vi "Read.vi"(6 "Timeout ms (1000)":i32=1000, 8 "Error In":errorcluster, 11 "Receiver Ref.":refnum<class "Receiver.lvclass">) -> (0 "Error Out":errorcluster, 1 "Received?":bool, 2 "Value":variant, 3 "Receiver Ref.":refnum<class "Receiver.lvclass">)   [LabVIEW 2020, in "RemoteVariables.lvlib" / "Receiver.lvclass"]
uses:
  Receiver.lvclass
  Receiver.lvclass/Receiver.ctl
  RawData.ctl
  RemoteVariables.lvlib
  UDP/UDP.lvclass
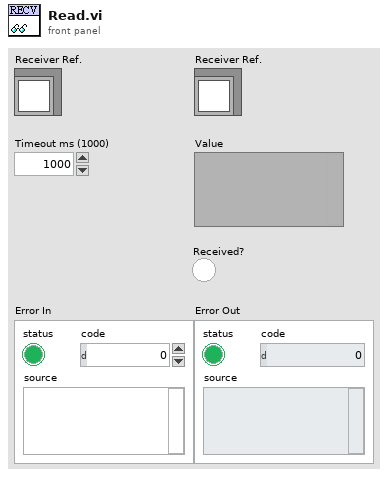
[diagram p1: front panel]
types:
  T1 = typedef "RemoteVariables.lvlib/RawData.ctl" = cluster{"Type string":i16[], "Data string":string}
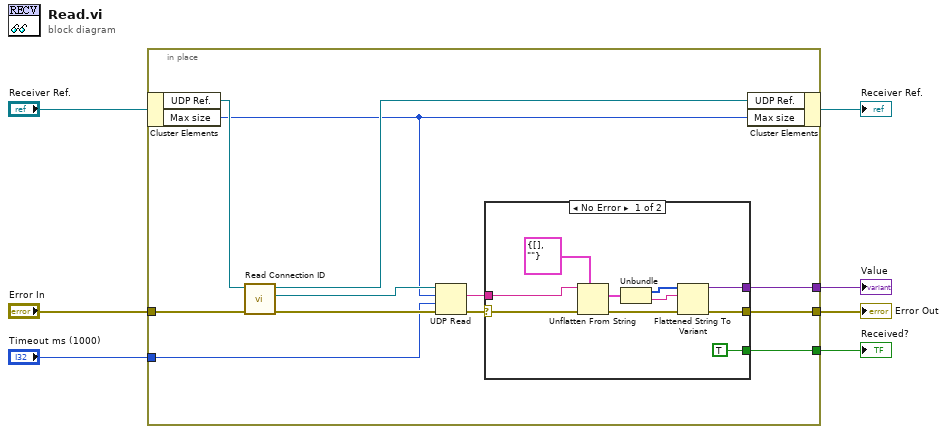
[diagram p0: block diagram]
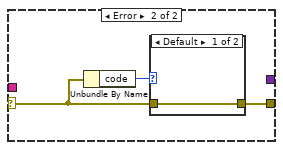
[diagram p2: hidden frame]
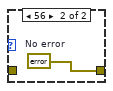
[diagram p3: hidden frame]
diagram:
  n1 = in-place {
    in-place-border: "Timeout ms (1000)" -> [w18]
    in-place-border: [w17] -> w6
    in-place-border: [w16] -> w5
    in-place-border: [w15] -> w4
    in-place-border: "Error In" -> [w12]
    n2 = in-place-cluster #1("Receiver Ref.") -> ("UDP Ref."=w10:refnum<class "UDP.lvclass">, "Max size"=w8:i32)
    n3 = call "Read Connection ID.vi"("error in (no error)"=w12, "UDP in"=w10) -> ("error out"=w19:errorcluster, "UDP Connection ID"=w11:refnum<k16>, "UDP out"=w9:refnum<class "UDP.lvclass">)  [unwired: 7 in]
    n4 = UDP Read(connection ID=w11, max size (548)=w8, timeout ms (25000)=w18, 8:w19) -> (data out=w13:string, error out=w14:errorcluster)  [unwired: 3 out]
    n5 = case shown="No Error" w14 {
      selector: w14 -> [w29 w31]
      tunnel: w13 -> [w28 _]
      tunnel: [w22 w30] -> w17
      tunnel: [w21 _] -> w16
      tunnel: [TRUE _] -> w15
      frame No Error {
        n6 = Unflatten From String(type=T1 {"Type string"=[], "Data string"=""} ("RawData"), binary string=w28, error in (no error)=w29) -> (value=w25:T1, error out=w26:errorcluster)  [unwired: 2 in, 1 out]
        n7 = Unbundle(w25) -> ("Type string"=w24:i16[], "Data string"=w23:string)
        n8 = Flattened String To Variant(4:w26, 6:w23, 7:w24) -> (0:w22:errorcluster, 3:w21:variant)
      }
      frame Error {
        n9 = Unbundle By Name(w31) -> ("code"=w32:i32)
        n10 = case shown="Default" w32 {
          tunnel: w31 -> [w33 _]
          tunnel: [w33 w34] -> w30
          frame Default {
          }
          frame 56 {
            w34 = errorcluster {"status"=FALSE, "code"=0, "source"=""}  # No error
          }
        }
      }
    }
    n11 = in-place-cluster #1("UDP Ref."=w9, "Max size"=w8) -> (→"Receiver Ref.":refnum<class "Receiver.lvclass">)
  }
  "Error Out" <- w6
  "Value" <- w5
  "Received?" <- w4
